vi "BRig_dataRT_stats__BTPR_avg_L.vi"() -> (2 "output_BTPR_avg_L__x100":i32)   [LabVIEW 2014]
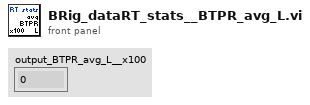
[diagram p1: front panel]
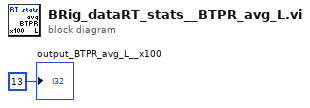
[diagram p0: block diagram]
diagram:
  "output_BTPR_avg_L__x100" <- 13 ("output_iBlock")
